vi "Initialize.vi"(4 "Y通道":string, 6 "X通道":string, 7 "原始采样率[Hz]":i32, 8 "error in (no error)":errorcluster caption="错误输入（无错误）", 9 "引用":T1, 10 "显示采样率[Hz]":i32, 11 "XYPlot 输入":refnum<class "TrendPlot.lvclass">) -> (0 "error out":errorcluster caption="错误输出", 3 "XYPlot 输出":refnum<class "TrendPlot.lvclass">)   [LabVIEW 2018, in "DataDisplay.lvlib" / "TrendPlot.lvclass"]
uses:
  TrendPlot.lvclass
  TrendPlotRef.vi
  TypeDefine/DD_DataStream.ctl
  <vilib>/Utility/miscctls.llb/LVPointTypeDef.ctl
  TypeDefine/DD_Command.ctl
  TrendPlot.lvclass/TrendPlot.ctl
  DataDisplay.lvlib
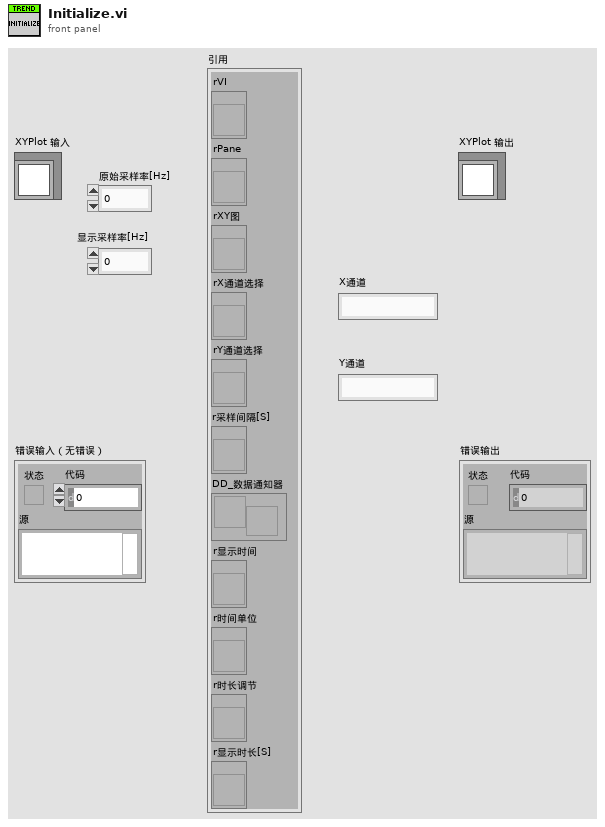
[diagram p1: front panel]
types:
  T1 = typedef "DataDisplay.lvlib/TrendPlot.lvclass/TrendPlotRef.vi" = cluster{"rVI":refnum<vi>, "rPane":refnum<vi>, "rXY图":refnum<vi>, "rX通道选择":refnum<vi>, "rY通道选择":refnum<vi>, "r采样间隔[S]":refnum<vi>, "DD_数据通知器":refnum<notifier>, "r显示时间":refnum<vi>, "r时间单位":refnum<vi>, "r时长调节":refnum<vi>, "r显示时长[S]":refnum<vi>}
  T2 = typedef "DataDisplay.lvlib/DD_Command.ctl" = cluster{"消息":string, "参数":variant}
  T3 = typedef "LVPointTypeDef.ctl" = cluster{"Horizontal":i16, "Vertical":i16}
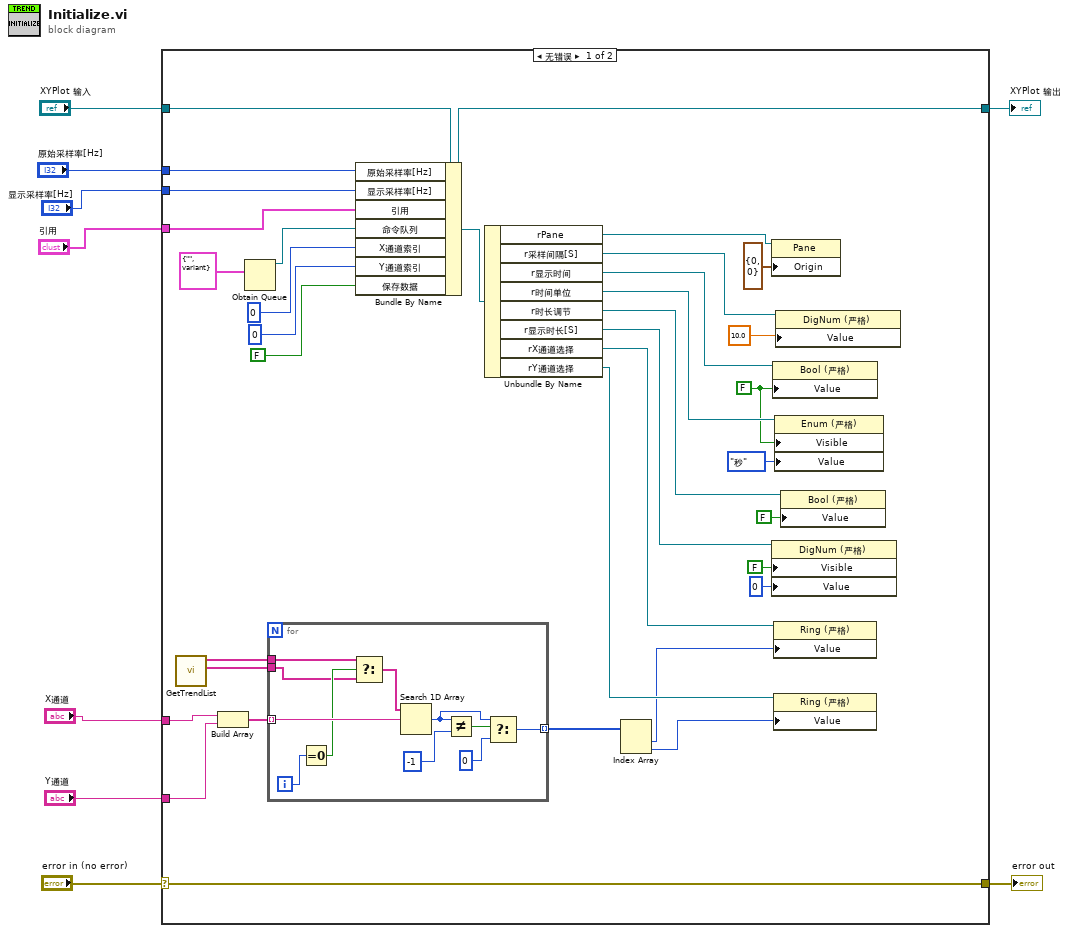
[diagram p0: block diagram]
diagram:
  n1 = case shown="无错误" "error in (no error)" {
    selector: "error in (no error)" -> [w42 w56]
    tunnel: [w42 w56] -> w8
    tunnel: [w41 w55] -> w6
    tunnel: "XYPlot 输入" -> [w43 w55]
    tunnel: "显示采样率[Hz]" -> [w40 _]
    tunnel: "引用" -> [w37 _]
    tunnel: "原始采样率[Hz]" -> [w32 _]
    tunnel: "X通道" -> [w13 _]
    tunnel: "Y通道" -> [w12 _]
    frame No Error {
      w27 = FALSE ("值")
      n2 = call "GetTrendList.vi"() -> ("Y列表"=w10:string[], "X列表"=w11:string[])  [unwired: 10 in]
      n3 = Build Array(w13, w12) -> (w14:string[])
      n4 = Obtain Queue(element data type=T2 {"消息"="", "参数"=variant} ("命令")) -> (queue out=w33:refnum<queue>)  [unwired: 4 in, 2 out]
      n5 = for {
        tunnel: [w50] -> w17 mode=indexing
        tunnel: w14 -> [w49] mode=indexing
        tunnel: w11 -> [w46]
        tunnel: w10 -> [w45]
        i -> [w48]
        n6 = Equal To 0?(x=w48) -> (x = 0?=w47:bool)
        n7 = Select(t=w46, s=w47, f=w45) -> (s? t:f=w44:string[])
        n8 = Search 1D Array(1D array=w44, element=w49) -> (index of element=w52:i32)  [unwired: 1 in]
        n9 = Not Equal?(x=w52, y=-1) -> (x != y?=w53:bool)
        n10 = Select(t=w52, s=w53, f=0) -> (s? t:f=w50:i32)
      }
      n11 = Bundle By Name(cluster=w43, "原始采样率[Hz]"=w32, "显示采样率[Hz]"=w40, "引用"=w37, "命令队列"=w33, "X通道索引"=0, "Y通道索引"=0, "保存数据"=FALSE) -> (w41:refnum<class "TrendPlot.lvclass">)
      n12 = Unbundle By Name(w41) -> ("rPane"=w39:refnum<vi>, "r采样间隔[S]"=w35:refnum<vi>, "r显示时间"=w29:refnum<vi>, "r时间单位"=w28:refnum<vi>, "r时长调节"=w25:refnum<vi>, "r显示时长[S]"=w23:refnum<vi>, "rX通道选择"=w19:refnum<vi>, "rY通道选择"=w18:refnum<vi>)
      n13 = Index Array(array=w17) -> (element #1=w16:i32, element #2=w15:i32)  [unwired: 2 in]
      n14 = property class="Pane"(reference=w39, "Origin"=T3 {"Horizontal"=0, "Vertical"=0} ("原点")) -> ()  [unwired: 1 in, 2 out]
      n15 = property class="DigNum (严格)"(reference=w23, "Visible"=FALSE ("可见"), "Value"=0 ("值")) -> ()  [unwired: 1 in, 2 out]
      n16 = property class="Bool (严格)"(reference=w29, "Value"=w27) -> ()  [unwired: 1 in, 2 out]
      n17 = property class="Ring (严格)"(reference=w19, "Value"=w16) -> ()  [unwired: 1 in, 2 out]
      n18 = property class="Ring (严格)"(reference=w18, "Value"=w15) -> ()  [unwired: 1 in, 2 out]
      n19 = property class="Enum (严格)"(reference=w28, "Visible"=w27, "Value"=enum16{"秒", "分钟", "小时"}."秒" ("值")) -> ()  [unwired: 1 in, 2 out]
      n20 = property class="DigNum (严格)"(reference=w35, "Value"=10.0 ("值")) -> ()  [unwired: 1 in, 2 out]
      n21 = property class="Bool (严格)"(reference=w25, "Value"=FALSE ("值")) -> ()  [unwired: 1 in, 2 out]
    }
    frame Error {
    }
  }
  "error out" <- w8
  "XYPlot 输出" <- w6
